vi "LEP_RV_ASW_GeneralTab.vi"(8 "error in (no error)":errorcluster, 10 "page sync rendezvous":T2, 11 "Close Event":refnum<user-event>) -> ()   [LabVIEW 2011]
uses:
  resource/dialog/PreferencesDialog/optionsFrame_EventData1.ctl
  <vilib>/LabVIEW Targets/Embedded/ASWServer/MPU_ASWServer_GeneralIcons.ctl
panel:
  out "Advance Progress Bar":bool
  in  "Progress Bar Steps":u32
  in  "Application Name Icon":T1
  in  "Target Name Icon":T1
  in  "Target Type Icon":T1
  in  "Download Status Icon":T1
  in  "Build Status Icon":T1
  out "cancel pressed?":bool
  out "Progress Bar Title":string="Unknown"
  out "Progress Bar":u32(slide) scale=0.0..100.0
  in  "Cancel":bool
  out "Application Name Pic":picture
  out "Target Name Pic":picture
  out "Download Status":string="Unknown"
  out "Application Name":string="Unknown"
  out "Build Status":string="Disconnected"
  out "Target Type":string="Unknown"
  out "Target Name":string="Unknown"
  out "Build Status Pic":picture
  out "Target Type Pic":picture
  out "Download Status Pic":picture
  in  "error msg format string":string="There was a problem applying the options from the %s category. The error message is \"%s.\""
  # "uVision Status:"
  # "Processor Status:"
  # "Exception Status:"
  # "Target Name:"
  # "Application Name:"
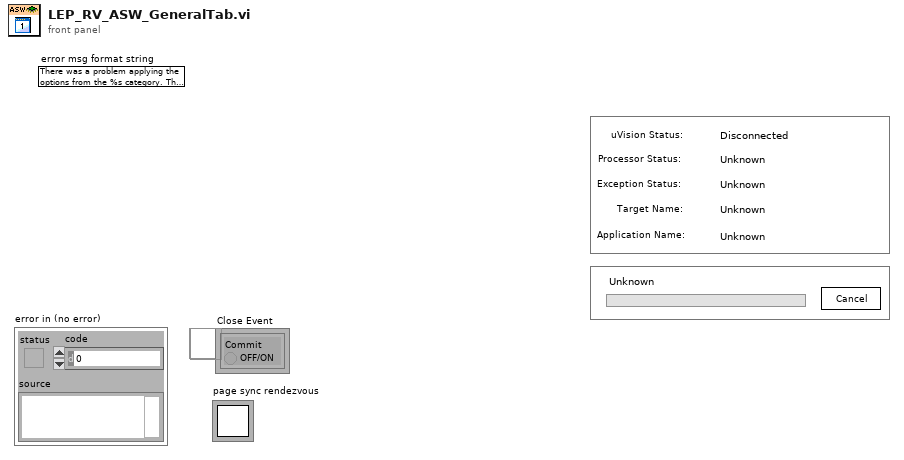
[diagram p1: front panel]
types:
  T1 = typedef "MPU_ASWServer_GeneralIcons.ctl" = enum16{"Complete", "Disconnected", "Error", "Initializing", "Ready", "Running", "Stopped", "Unknown", "No Change"}
  T2 = typedef "Rendezvous RefNum" = refnum<k1>
  T3 = enum8{"Enabled", "Disabled", "Disabled and Grayed Out"}
  T4 = typedef "imagedata.ctl" = cluster{"image type":i32, "image depth":i32, "image":u8[], "mask":u8[], "colors":u32[], "Rectangle":cluster{"left":i16, "top":i16, "right":i16, "bottom":i16}}
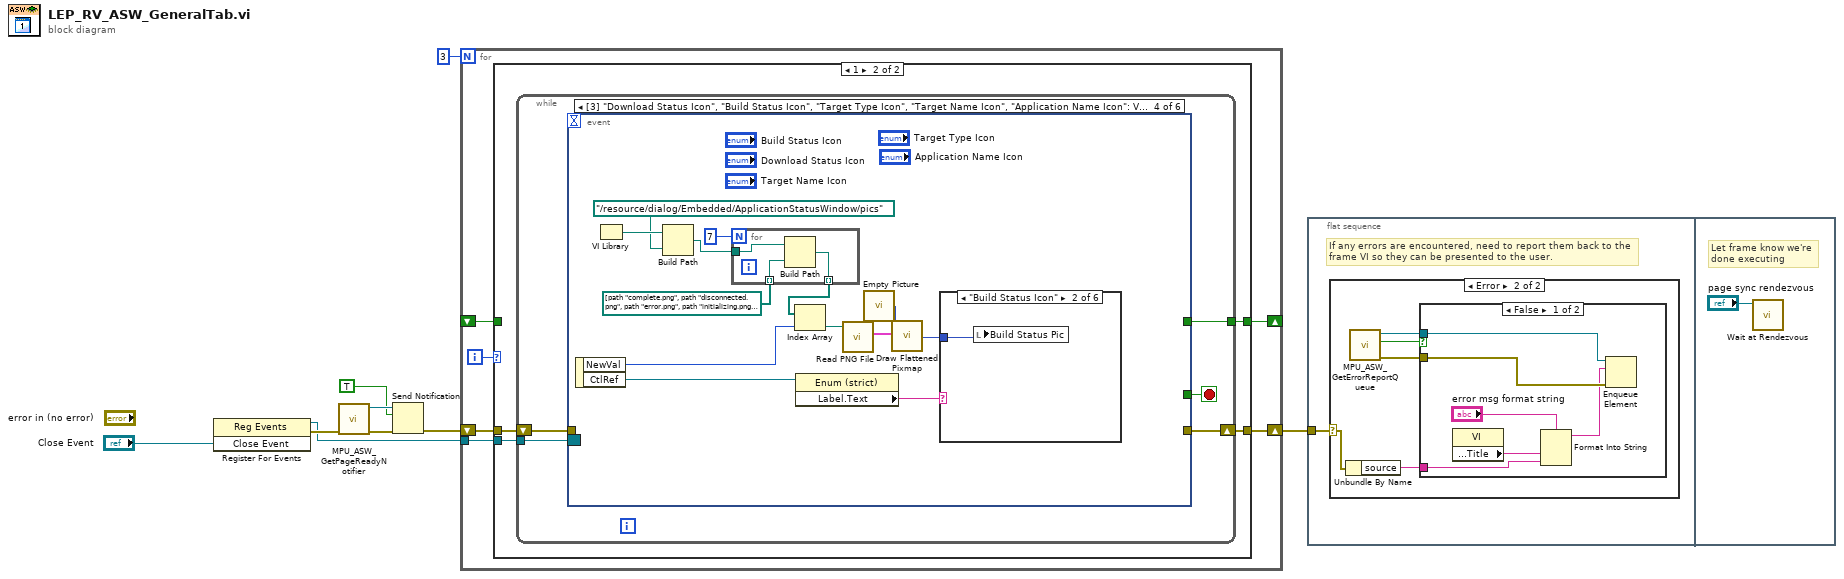
[diagram p0: block diagram]
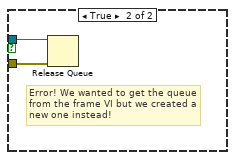
[diagram p3: hidden frame]
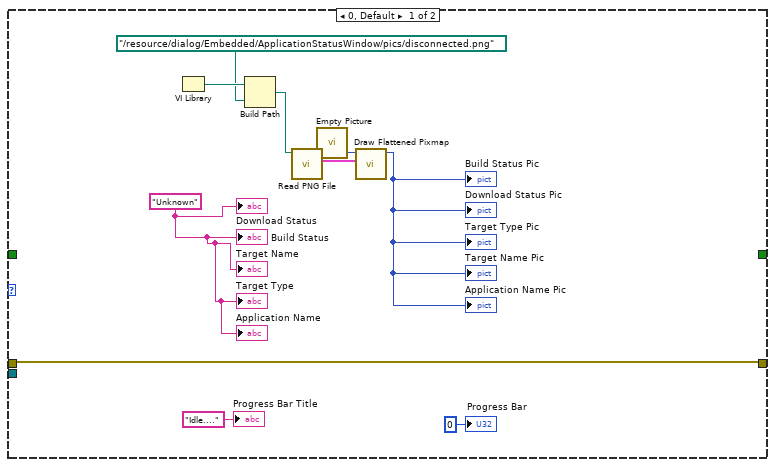
[diagram p4: hidden frame]
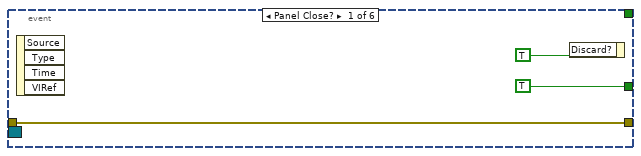
[diagram p5: hidden frame]
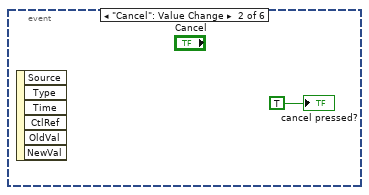
[diagram p6: hidden frame]
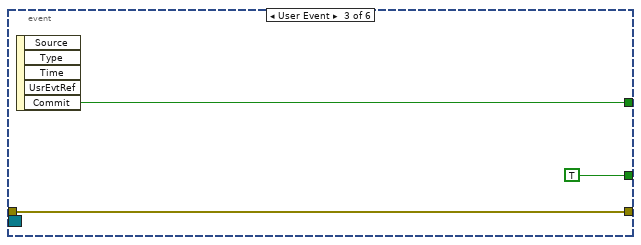
[diagram p7: hidden frame]
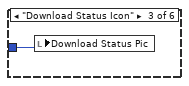
[diagram p9: hidden frame]
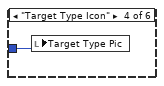
[diagram p10: hidden frame]
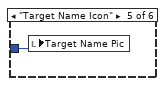
[diagram p11: hidden frame]
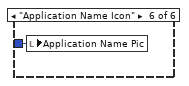
[diagram p12: hidden frame]
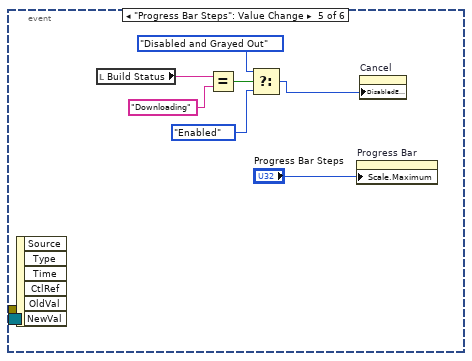
[diagram p13: hidden frame]
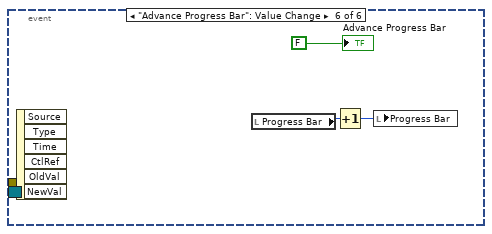
[diagram p14: hidden frame]
diagram:
  n1 = register-events("Close Event") -> (reference out=w4:refnum<event-registration>, error out=w6:errorcluster)  [unwired: 2 in]
  n2 = call "MPU_ASW_GetPageReadyNotifier.vi"("error in (no error)"=w6) -> ("error out"=w8:errorcluster, "notifier out"=w9:refnum<notifier>)  [unwired: 9 out]
  n3 = Send Notification(notification=TRUE, notifier=w9, error in (no error)=w8) -> (error out=w2:errorcluster)  [unwired: 1 out]
  n4 = for {
    N: 3 -> [_]
    shift-right: [w10] -> w3
    shift-left: w2 -> [w14]
    shift-right: [w13] -> _
    shift-left: _ -> [w12]
    tunnel: w4 -> [w11]
    i -> [w15]
    n5 = case shown="1" w15 {
      tunnel: w14 -> [w25 w29]
      tunnel: [_ w26] -> w13
      tunnel: w12 -> [_ _]
      tunnel: w11 -> [_ w28]
      tunnel: [w25 w27] -> w10
      frame 0, Default {
        w19 = "Unknown" ("Download Status")
        n6 = VI Library() -> (path=w18:path)
        n7 = Build Path(base path=w18, name or relative path=path "../resource/dialog/Embedded/ApplicationStatusWindow/pics/disconnected.png") -> (appended path=w16:path)
        n8 = call <vilib>:"Read PNG File.vi"("path to PNG file"=w16) -> ("image data"=w24:T4)  [unwired: 1 in, 9 out]
        n9 = call "Empty Picture"() -> ("empty picture"=w23:picture)
        n10 = call <vilib>:"Draw Flattened Pixmap.vi"("image data"=w24, "picture"=w23) -> ("new picture"=→"Download Status Pic" →"Target Type Pic" →"Build Status Pic" →"Target Name Pic" →"Application Name Pic":picture)  [unwired: 7 out]
        "Target Type" <- w19
        "Build Status" <- w19
        "Application Name" <- w19
        "Download Status" <- w19
        "Target Name" <- w19
        "Progress Bar Title" <- "Idle...." ("Progress Bar Title")
        "Progress Bar" <- u8 0 ("ProgressBar")
      }
      frame 1 {
        n11 = while {
          shift-right: [w33] -> w27
          shift-left: w29 -> [w34]
          tunnel: [w32] -> w26
          tunnel: w28 -> [w30]
          stop <- w31 stop-if-true
          n12 = event shown="[3] \"Download Status Icon\", \"Build Status Icon\", \"Target Type Icon\", \"Target Name Icon\", \"Application Name Icon\": Value Change" {
            selector: w30 -> [_ _ _ _ _ _]
            dyn-events: _ -> [_ _ _ _ _ _]
            timeout: _ -> [_ _ _ _ _ _]
            tunnel: w34 -> [w36 _ w39 _ _ _]
            tunnel: [w36 _ w39 _ _ _] -> w33
            tunnel: [_ _ w41 _ _ _] -> w32
            tunnel: [TRUE _ TRUE _ _ _] -> w31
            event Panel Close? {
              n13 = event-data() -> ()  [unwired: 5 out]
              n14 = event-data("Discard?"=TRUE) -> ()  [unwired: 1 in, 1 out]
            }
            event "Cancel": Value Change {
              n15 = event-data() -> ()  [unwired: 7 out]
              "cancel pressed?" <- TRUE ("cancel pressed?")
            }
            event User Event {
              n16 = event-data() -> ("Commit"=w41:bool)  [unwired: 5 out]
            }
            event Value Change {
              n17 = event-data() -> ("NewVal"=w52:T1, "CtlRef"=w54:refnum<vi>)  [unwired: 1 out]
              n18 = VI Library() -> (path=w46:path)
              n19 = Build Path(base path=w46, name or relative path=path "../resource/dialog/Embedded/ApplicationStatusWindow/pics") -> (appended path=w45:path)
              n20 = for {
                N: 7 -> [_]
                tunnel: w45 -> [w56]
                tunnel: path[] [path "complete.png", path "disconnected.png", path "error.png", path "initializing.png", path "ready.png", path "running.png", path "stopped.png", path "unknown.png"] -> [w57] mode=indexing
                tunnel: [w55] -> w42 mode=indexing
                n21 = Build Path(base path=w56, name or relative path=w57) -> (appended path=w55:path)
              }
              n22 = Index Array(array=w42, index=w52) -> (element=w51:path)
              n23 = property class="Enum (strict)"(reference=w54) -> ("Label.Text"=w53:string)  [unwired: 1 in, 2 out]
              n24 = call <vilib>:"Read PNG File.vi"("path to PNG file"=w51) -> ("image data"=w50:T4)  [unwired: 1 in, 9 out]
              n25 = call "Empty Picture"() -> ("empty picture"=w49:picture)
              n26 = call <vilib>:"Draw Flattened Pixmap.vi"("image data"=w50, "picture"=w49) -> ("new picture"=w48:picture)  [unwired: 7 out]
              n27 = case shown="\"Build Status Icon\"" w53 {
                tunnel: w48 -> [_ w58 w59 w60 w61 w62]
                frame Default {
                }
                frame "Build Status Icon" {
                  n28 = local write "Build Status Pic"(w58) -> ()
                }
                frame "Download Status Icon" {
                  n29 = local write "Download Status Pic"(w59) -> ()
                }
                frame "Target Type Icon" {
                  n30 = local write "Target Type Pic"(w60) -> ()
                }
                frame "Target Name Icon" {
                  n31 = local write "Target Name Pic"(w61) -> ()
                }
                frame "Application Name Icon" {
                  n32 = local write "Application Name Pic"(w62) -> ()
                }
              }
            }
            event "Progress Bar Steps": Value Change {
              n33 = event-data() -> ()  [unwired: 7 out]
              n34 = local read "Build Status"() -> (w68:string)
              n35 = Equal?(x=w68, y="Downloading") -> (x = y?=w67:bool)
              n36 = Select(t=T3."Disabled and Grayed Out" ("Disabled"), s=w67, f=T3."Enabled") -> (s? t:f=w64:T3)
              n37 = property on="Progress Bar" class="Slide (strict)"("Scale.Maximum"="Progress Bar Steps") -> ()  [unwired: 2 in, 2 out]
              n38 = property on="Cancel" class="Bool"("DisabledEnum"=w64) -> ()  [unwired: 2 in, 2 out]
            }
            event "Advance Progress Bar": Value Change {
              n39 = event-data() -> ()  [unwired: 7 out]
              n40 = local read "Progress Bar"() -> (w70:u32)
              n41 = Increment(x=w70) -> (x+1=w71:u32)
              n42 = local write "Progress Bar"(w71) -> ()
              "Advance Progress Bar" <- FALSE ("Advance Progress Bar")
            }
          }
        }
      }
    }
  }
  n43 = flat-sequence {
    tunnel: w3 -> [w73]
    frame #0 {
      # "If any errors are encountered, need to report them back to the \nframe VI so they can be presented to the user."
      n44 = case shown="Error" w73 {
        selector: w73 -> [_ w75]
        frame No Error {
        }
        frame Error {
          n45 = Unbundle By Name(w75) -> ("source"=w74:string)
          n46 = call "MPU_ASW_GetErrorReportQueue.vi"() -> ("error out"=w76:errorcluster, "created new?"=w78:bool, "queue out"=w77:refnum<queue>)  [unwired: 9 out]
          n47 = case shown="False" w78 {
            tunnel: w77 -> [w84 w86]
            tunnel: w76 -> [w83 w85]
            tunnel: w74 -> [w80 _]
            frame False {
              n48 = property class="VI"() -> ("Front Panel.Title"=w81:string)  [unwired: 2 in, 2 out]
              n49 = Format Into String(format string="error msg format string", w81, w80) -> (resulting string=w79:string)  [unwired: 2 in, 1 out]
              n50 = Enqueue Element(queue=w84, element=w79, error in (no error)=w83) -> ()  [unwired: 4 out]
            }
            frame True {
              # "Error! We wanted to get the queue\nfrom the frame VI but we created a\nnew one instead!"
              n51 = Release Queue(queue=w86, error in (no error)=w85) -> ()  [unwired: 4 out]
            }
          }
        }
      }
    }
    frame #1 {
      # "Let frame know we're \ndone executing"
      n52 = call <vilib>:"Wait at Rendezvous.vi"("rendezvous"="page sync rendezvous") -> ()  [unwired: 2 in, 5 out]
    }
  }
